vi "ContinousLoopMain.vi"() -> ()   [LabVIEW 2018]
uses:
  <userlib>/Tango_DLL/Tango_DLL.lvlib
  lib/Olympus IX BX Series/Olympus IX BX Series.lvlib
panel:
  out "queue out":refnum<queue>
  out "error out":errorcluster
  out "Interval":timestamp format="%<%X\n%x>T"
  out "Total Duration":timestamp format="%<%X\n%x>T"
  out "File Prefix":string
  out "SaveDir":path
  out "Intensity":dbl[](array[numeric])
  out "Prism":string[](array[string])
  out "Exposure Time":i32[](array[numeric])
  out "Filter":string[](array[string])
  out "Objective":i32[](array[numeric])
  in  "Load file":bool
  in  "Start Program":bool
  in  "stop":bool
  out "Positions":dbl[][](array[numeric])
  in  "Load Configuration File":path=path "C:/Users/johan/Downloads/LabVIEW software/LabVIEW software/IX-81 Software/Config_Files/191119_config_surface.xml"
  out "Continuous Program":string[][](array[string])
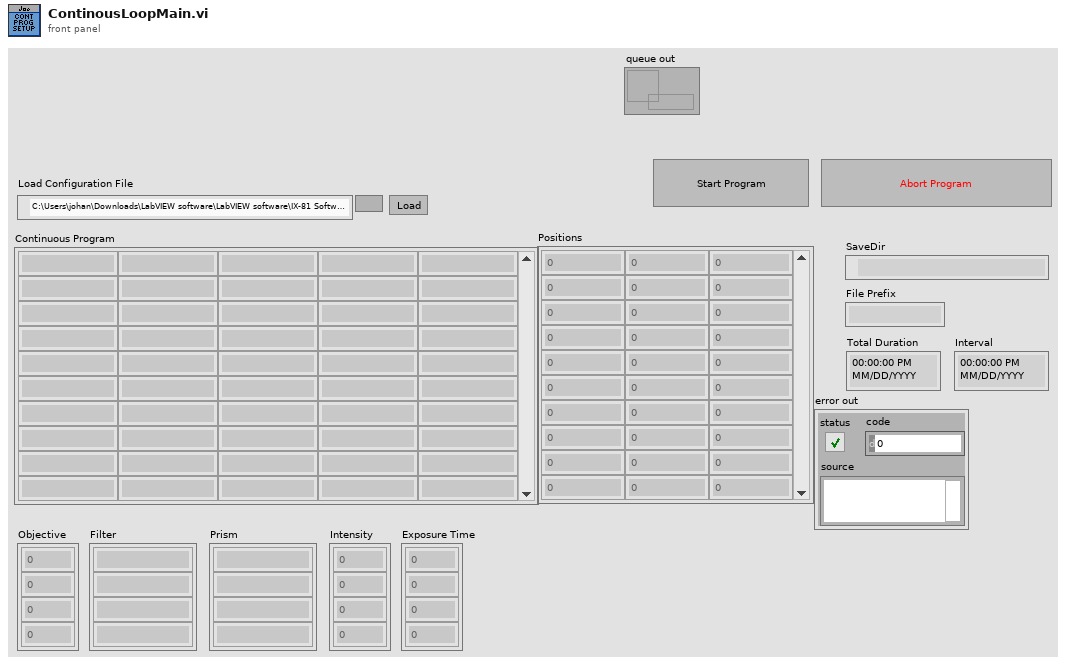
[diagram p1: front panel]
types:
  T1 = enum8{"Enabled", "Disabled", "Disabled and Grayed Out"}
  T2 = cluster{"Step Name":string, "Time":timestamp, "Param 1":dbl, "Param 2":i32}
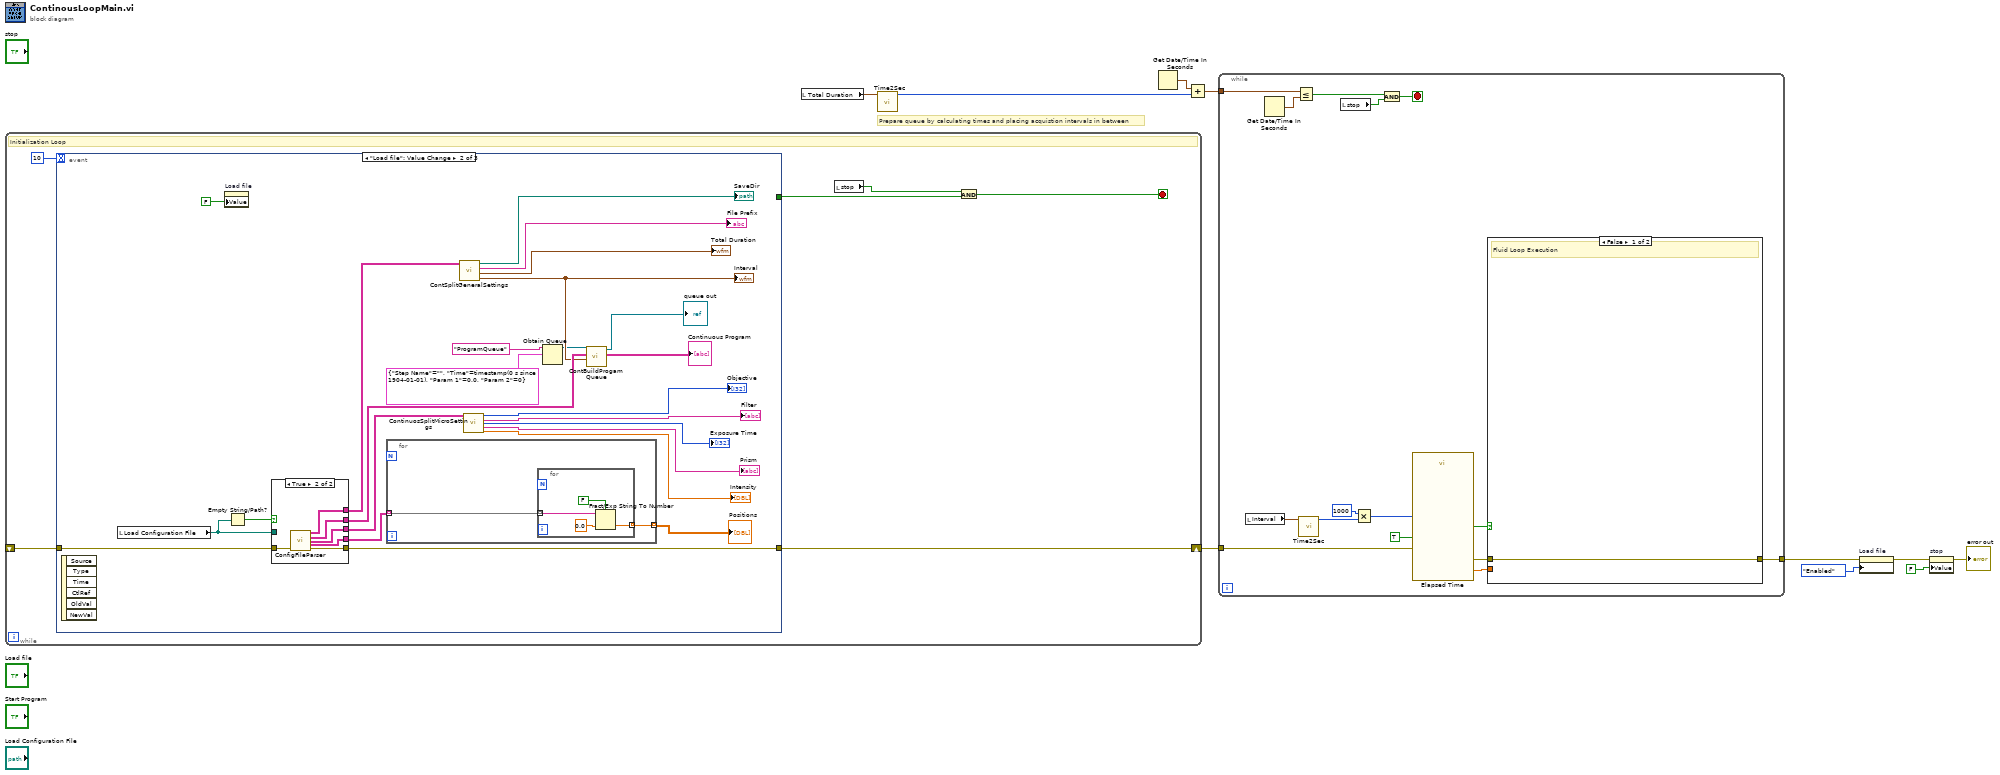
[diagram p0: block diagram]
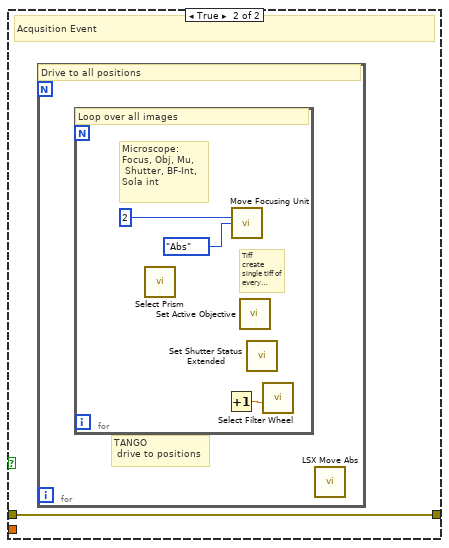
[diagram p2: hidden frame]
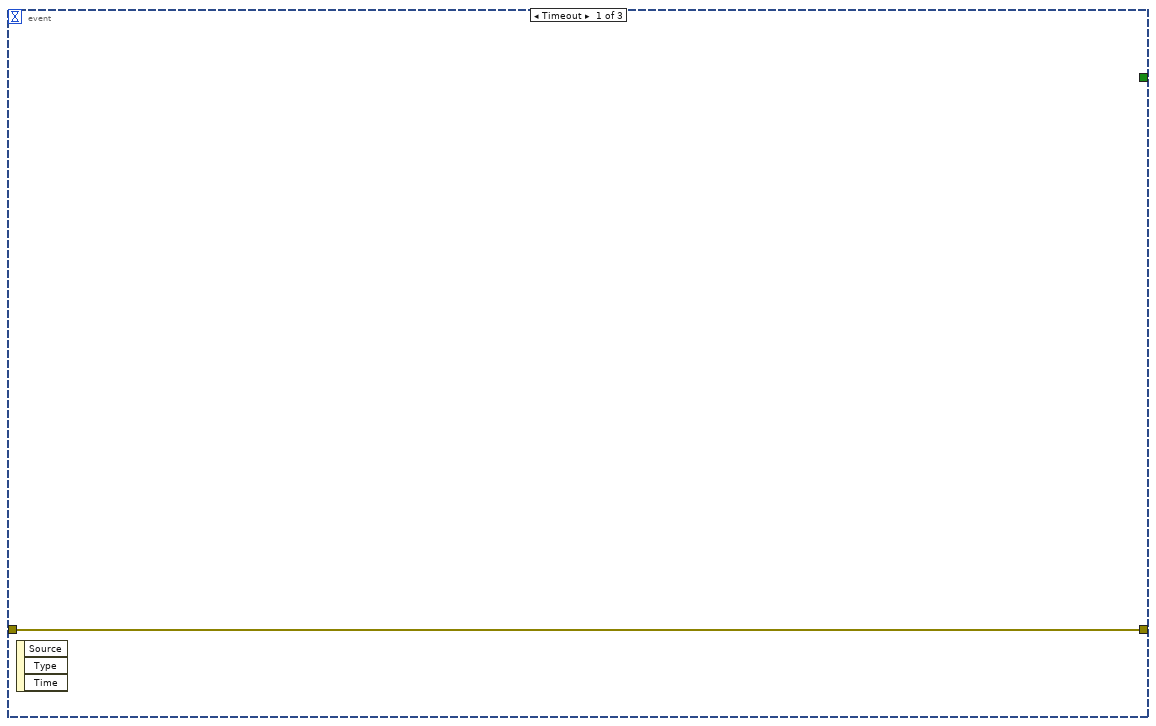
[diagram p3: hidden frame]
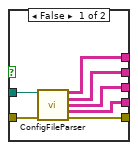
[diagram p4: hidden frame]
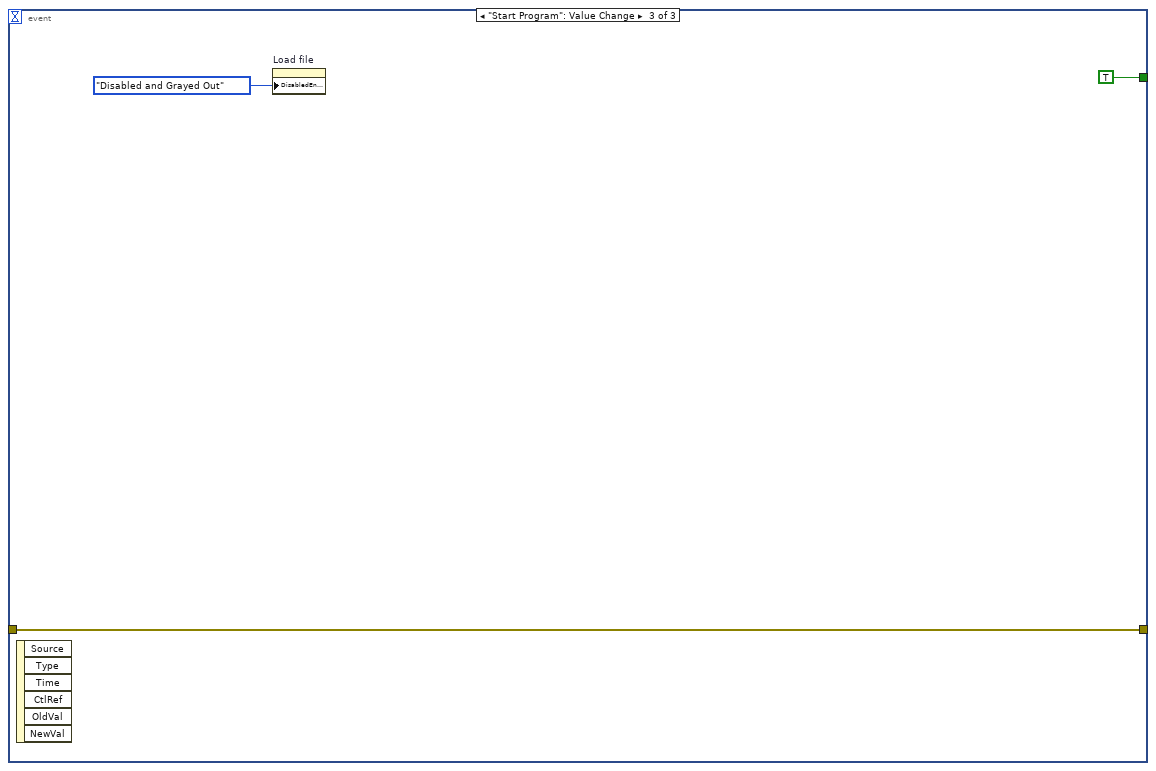
[diagram p5: hidden frame]
diagram:
  # "Prepare queue by calculating times and placing acquistion intervals in between"
  n1 = while {
    shift-right: [w12] -> w4
    shift-left: _ -> [w11]
    stop <- w15 stop-if-true
    # "Initialization Loop"
    n2 = event shown="[1] \"Load file\": Value Change" {
      selector: _ -> [_ _ _]
      dyn-events: _ -> [_ _ _]
      timeout: 10 -> [_ _ _]
      tunnel: [_ _ TRUE] -> w14
      tunnel: [w17 w24 w61] -> w12
      tunnel: w11 -> [w17 w23 w61]
      event Timeout {
        n3 = event-data() -> ()  [unwired: 1 in, 3 out]
      }
      event "Load file": Value Change {
        n4 = event-data() -> ()  [unwired: 1 in, 6 out]
        n5 = local read "Load Configuration File"() -> (w38:path)
        n6 = property on="Load file" class="Bool (strict)"("Value"=FALSE ("Load file")) -> ()  [unwired: 2 in, 2 out]
        n7 = Empty String/Path?(string/path=w38) -> (empty?=w39:bool)
        n8 = case shown="True" w39 {
          tunnel: w38 -> [w54 _]
          tunnel: [w53 w60] -> w26
          tunnel: [w52 w58] -> w40
          tunnel: [w51 w59] -> w36
          tunnel: [w50 w57] -> w30
          tunnel: [w49 w56] -> w24
          tunnel: w23 -> [w48 w55]
          frame False {
            n9 = call "ConfigFileParser.vi"("Path"=w54, "error in"=w48) -> ("General Settings"=w50:string[][], "Program"=w53:string[][], "Loop Microscope Settings"=w51:string[][], "Positions"=w52:string[][], "error out"=w49:errorcluster)  [unwired: 8 in, 1 out]
          }
          frame True {
            n10 = call "ConfigFileParser.vi"("error in"=w55) -> ("General Settings"=w57:string[][], "Program"=w60:string[][], "Loop Microscope Settings"=w59:string[][], "Positions"=w58:string[][], "error out"=w56:errorcluster)  [unwired: 9 in, 1 out]
          }
        }
        n11 = for {
          tunnel: w40 -> [w43] mode=indexing
          tunnel: [w42] -> w41 mode=indexing
          n12 = for {
            tunnel: w43 -> [w47] mode=indexing
            tunnel: [w46] -> w42 mode=indexing
            n13 = Fract/Exp String To Number(use system decimal point (T)=FALSE, string=w47, default (0 dbl)=0.0 ("default (0 DBL)")) -> (number=w46:dbl)  [unwired: 1 in, 1 out]
          }
        }
        "Positions" <- w41
        n14 = call "ContSplitGeneralSettings.vi"("General Settings"=w30) -> ("Interval"=w22:timestamp, "Total Duration"=→"Total Duration":timestamp, "File Prefix"=→"File Prefix":string, "SaveDir"=→"SaveDir":path)  [unwired: 7 in]
        "Interval" <- w22
        n15 = call "ContinuosSplitMicroSettings.vi"("Loop Microscope Settings"=w36) -> ("Objective"=→"Objective":i32[], "Filter"=→"Filter":string[], "Exposure Time"=→"Exposure Time":i32[], "Prism"=→"Prism":string[], "Intensity"=→"Intensity":dbl[])  [unwired: 10 in]
        n16 = Obtain Queue(name (unnamed)="ProgramQueue", element data type=T2 {"Step Name"="", "Time"=timestamp(0 s since 1904-01-01), "Param 1"=0.0, "Param 2"=0}) -> (queue out=w19:refnum<queue>)  [unwired: 3 in, 2 out]
        n17 = call "ContBuildProgamQueue.vi"("Acquisition Interval"=w22, "Continuous Program"=w26, "queue în"=w19) -> ("Continuous Program modified"=→"Continuous Program":string[][], "queue out"=→"queue out":refnum<queue>)  [unwired: 7 in]
      }
      event "Start Program": Value Change {
        n18 = event-data() -> ()  [unwired: 1 in, 6 out]
        n19 = property on="Load file" class="Bool (strict)"("DisabledEnum"=T1."Disabled and Grayed Out" ("Disabled")) -> ()  [unwired: 2 in, 2 out]
      }
    }
    n20 = local read "stop"() -> (w13:bool)
    n21 = And(x=w13, y=w14) -> (x .and. y?=w15:bool)
  }
  n22 = local read "Total Duration"() -> (w8:timestamp)
  n23 = call "Time2Sec.vi"("Total Duration"=w8) -> ("Numeric"=w6:i32)  [unwired: 10 in]
  n24 = Get Date/Time In Seconds() -> (seconds since 1Jan1904=w7:timestamp)
  n25 = Add(x=w7, y=w6) -> (x+y=w5:timestamp)
  n26 = while {
    tunnel: w5 -> [w76]
    tunnel: w4 -> [w67]
    tunnel: [w65] -> w3
    stop <- w75 stop-if-true
    n27 = local read "Interval"() -> (w70:timestamp)
    n28 = Get Date/Time In Seconds() -> (seconds since 1Jan1904=w77:timestamp)
    n29 = Less Or Equal?(x=w76, y=w77) -> (x <= y?=w74:bool)
    n30 = call "Time2Sec.vi"("Total Duration"=w70) -> ("Numeric"=w73:i32)  [unwired: 10 in]
    n31 = local read "stop"() -> (w78:bool)
    n32 = Multiply(x=1000, y=w73) -> (x*y=w69:i32)
    n33 = And(x=w74, y=w78) -> (x .and. y?=w75:bool)
    n34 = call "Elapsed Time"("Time Target (s)"=w69, "Auto Reset"=TRUE, "error in (no error)"=w67) -> ("Elapsed Time (s)"=w64:dbl, "Time has Elapsed"=w68:bool, "error out"=w66:errorcluster)  [unwired: 9 in, 5 out]
    n35 = case shown="False" w68 {
      tunnel: w66 -> [w79 w80]
      tunnel: [w79 w80] -> w65
      tunnel: w64 -> [_ _]
      frame False {
        # "Fluid Loop Execution"
      }
      frame True {
        # "Acqusition Event"
        n36 = for {
          # "TANGO\n drive to positions"
          # "Drive to all positions"
          n37 = for {
            # "Microscope: \nFocus, Obj, Mu,\n Shutter, BF-Int, \nSola int"
            # "Tiff\ncreate single tiff of every timestamp"
            # "Loop over all images"
            n38 = call "Select Prism.vi"() -> ()  [unwired: 10 in, 2 out]
            n39 = Increment() -> (x+1=w81:dbl)  [unwired: 1 in]
            n40 = call "Move Focusing Unit.vi"("Device Number (1)"=2, "Direction (1: Down)"=enum16{"Up", "Down", "Abs"}."Abs") -> ()  [unwired: 12 in, 2 out]
            n41 = call "Set Active Objective.vi"() -> ()  [unwired: 10 in, 2 out]
            n42 = call "Set Shutter Status Extended.vi"() -> ()  [unwired: 14 in, 2 out]
            n43 = call "Select Filter Wheel.vi"("Filter Wheel Position (1)"=w81) -> ()  [unwired: 9 in, 2 out]
          }
          n44 = call <userlib>:"LSX Move Abs.vi"() -> ()  [unwired: 10 in, 2 out]
        }
      }
    }
  }
  n45 = property on="Load file" class="Bool (strict)"(error in=w3, "DisabledEnum"=T1."Enabled" ("Disabled")) -> (error out=w2:errorcluster)  [unwired: 1 in, 1 out]
  n46 = property on="stop" class="Bool (strict)"(error in=w2, "Value"=FALSE ("stop")) -> (error out=→"error out":errorcluster)  [unwired: 1 in, 1 out]
